vi "calc_time.vi"(11 "start time":u32) -> (3 "String":string)   [LabVIEW 2020, in "librarian.lvclass"]
uses:
  librarian.lvclass
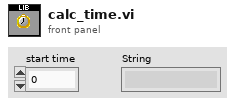
[diagram p1: front panel]
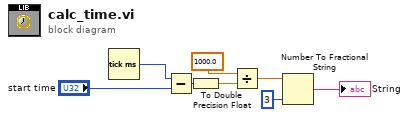
[diagram p0: block diagram]
diagram:
  n1 = Tick Count (ms)() -> (millisecond timer value=w1:u32)
  n2 = Subtract(x=w1, y="start time") -> (x-y=w3:u32)
  n3 = To Double Precision Float(number=w3) -> (double precision float=w5:dbl)
  n4 = Divide(x=1000.0, y=w5) -> (x/y=w6:dbl)
  n5 = Number To Fractional String(number=w6, precision (6)=i16 3) -> (F-format string=→"String":string)  [unwired: 2 in]
